vi "12_DC Motor_2.vi"() -> ()   [LabVIEW 2018]
uses:
  <userlib>/KNR OS 4.0 LabVIEW Toolkit/Type Definition/Resource.ctl
  <userlib>/KNR OS 4.0 LabVIEW Toolkit/Type Definition/DC Motor Port.ctl
panel:
  in  "Reset 2":bool
  in  "Reverse? 2":bool
  out "Velocity (cts/sec) 2":dbl
  out "Position 2":i32
  in  "Speed (+-100%) 2":dbl(slide) scale=-5.0..5.0
  in  "Enable Motor 2":bool
  in  "IP":string(combo)="172.22.11.2"
  in  "Resource":T1=enum."KNRm_DDDD"
  in  "stop":bool
  in  "Enable Motor":bool
  in  "Speed (+-100%)":dbl(slide) scale=-5.0..5.0
  out "Position":i32
  out "Velocity (cts/sec)":dbl
  in  "Reverse?":bool
  in  "Reset":bool
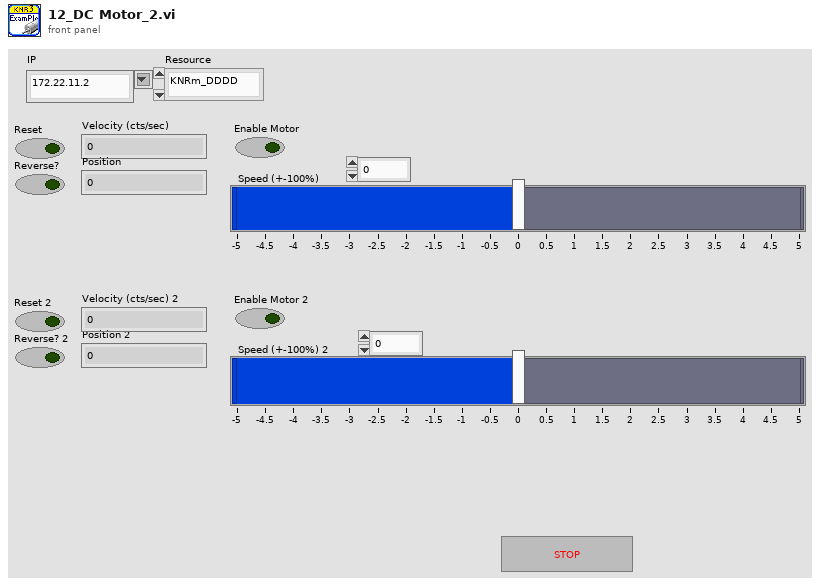
[diagram p1: front panel]
types:
  T1 = typedef "Resource.ctl" = enum16{"KNRm_DDRC", "KNRm_DDDD", "KNRm_DDDR", "KNRm_DDDC", "KNR", "KNRm_neww"}
  T2 = typedef "KNR3 Reference.ctl" = cluster{"FPGA Session":refnum<class "FPGA Interface Base.lvclass">, "Resource":T1}
  T3 = typedef "DC Motor Port.ctl" = u16
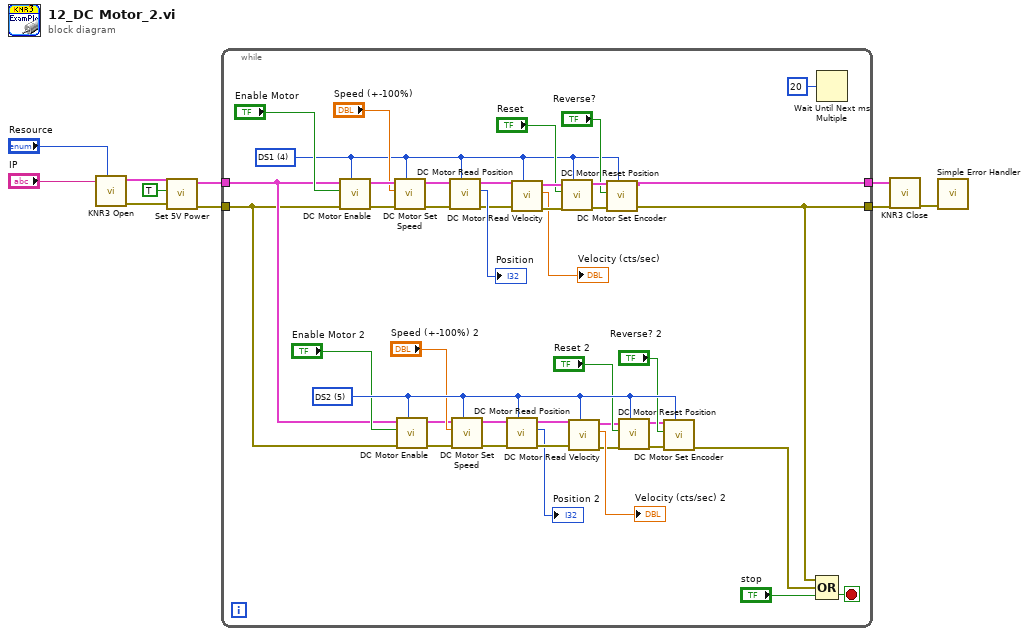
[diagram p0: block diagram]
diagram:
  n1 = call <userlib>:"KNR3 Open.vi"("Resource"="Resource", "IP"="IP") -> ("error out"=w2:errorcluster, "KNR out"=w4:T2)  [unwired: 8 in]
  n2 = call <userlib>:"Set 5V Power.vi"("error in (no error)"=w2, "5V Power(T)"=TRUE ("5V Power"), "KNR in"=w4) -> ("error out"=w8:errorcluster, "KNR out"=w9:T2)  [unwired: 7 in]
  n3 = while {
    tunnel: w9 -> [w14]
    tunnel: w8 -> [w13]
    tunnel: [w11] -> w6
    tunnel: [w38] -> w7
    stop <- w44 stop-if-true
    w31 = T3 5 items=["DS1"=4, "DS2"=5, "DS3"=6, "DS4"=7] ("Port")
    w32 = T3 4 items=["DS1"=4, "DS2"=5, "DS3"=6, "DS4"=7] ("Port")
    n4 = call <userlib>:"DC Motor Enable.vi"("Port (DS1)"=w32, "error in (no error)"=w13, "Enable Motor(F)"="Enable Motor", "KNR in"=w14) -> ("error out"=w47:errorcluster, "KNR out"=w52:T2)  [unwired: 6 in]
    n5 = call <userlib>:"DC Motor Set Speed.vi"("Port (DS1)"=w32, "error in (no error)"=w47, "Speed (+-100%)"="Speed (+-100%)", "KNR in"=w52) -> ("error out"=w46:errorcluster, "KNR out"=w51:T2)  [unwired: 6 in]
    n6 = call <userlib>:"DC Motor Enable.vi"("Port (DS1)"=w31, "error in (no error)"=w13, "Enable Motor(F)"="Enable Motor 2", "KNR in"=w14) -> ("error out"=w20:errorcluster, "KNR out"=w15:T2)  [unwired: 6 in]
    n7 = call <userlib>:"DC Motor Read Position.vi"("Port (DS1)"=w32, "error in (no error)"=w46, "KNR in"=w51) -> ("error out"=w41:errorcluster, "Position"=→"Position":i32, "KNR out"=w42:T2)  [unwired: 6 in]
    n8 = call <userlib>:"DC Motor Set Speed.vi"("Port (DS1)"=w31, "error in (no error)"=w20, "Speed (+-100%)"="Speed (+-100%) 2", "KNR in"=w15) -> ("error out"=w21:errorcluster, "KNR out"=w16:T2)  [unwired: 6 in]
    n9 = call <userlib>:"DC Motor Read Position.vi"("Port (DS1)"=w31, "error in (no error)"=w21, "KNR in"=w16) -> ("error out"=w23:errorcluster, "Position"=→"Position 2":i32, "KNR out"=w22:T2)  [unwired: 6 in]
    n10 = call <userlib>:"DC Motor Read Velocity.vi"("Port (DS1)"=w32, "error in (no error)"=w41, "KNR in"=w42) -> ("error out"=w36:errorcluster, "Velocity (cts/sec)"=→"Velocity (cts/sec)":dbl, "KNR out"=w40:T2)  [unwired: 6 in]
    n11 = call <userlib>:"DC Motor Reset Position.vi"("Port (DS1)"=w32, "error in (no error)"=w36, "Reset(F)"="Reset", "KNR in"=w40) -> ("error out"=w37:errorcluster, "KNR out"=w39:T2)  [unwired: 6 in]
    n12 = call <userlib>:"DC Motor Read Velocity.vi"("Port (DS1)"=w31, "error in (no error)"=w23, "KNR in"=w22) -> ("error out"=w27:errorcluster, "Velocity (cts/sec)"=→"Velocity (cts/sec) 2":dbl, "KNR out"=w24:T2)  [unwired: 6 in]
    n13 = call <userlib>:"DC Motor Set Encoder.vi"("Port (DS1)"=w32, "error in (no error)"=w37, "Reverse?(F)"="Reverse?", "KNR in"=w39) -> ("error out"=w11:errorcluster, "KNR out"=w38:T2)  [unwired: 6 in]
    n14 = call <userlib>:"DC Motor Reset Position.vi"("Port (DS1)"=w31, "error in (no error)"=w27, "Reset(F)"="Reset 2", "KNR in"=w24) -> ("error out"=w26:errorcluster, "KNR out"=w25:T2)  [unwired: 6 in]
    n15 = call <userlib>:"DC Motor Set Encoder.vi"("Port (DS1)"=w31, "error in (no error)"=w26, "Reverse?(F)"="Reverse? 2", "KNR in"=w25) -> ("error out"=w12:errorcluster)  [unwired: 6 in, 1 out]
    n16 = Compound Arithmetic op=OR(w11, w12, "stop") -> (w44:bool)
    n17 = Wait Until Next ms Multiple(millisecond multiple=u32 20) -> ()  [unwired: 1 out]
  }
  n18 = call <userlib>:"KNR3 Close.vi"("error in (no error)"=w6, "KNR in"=w7) -> ("error out"=w5:errorcluster)  [unwired: 9 in]
  n19 = call <vilib>:"Simple Error Handler.vi"("error in (no error)"=w5) -> ()  [unwired: 4 in, 5 out]
